vi "2_test_1.vi"() -> ()   [LabVIEW 2020]
uses:
  <vilib>/vision/driver/NI_Vision_Acquisition_Software.lvlib
panel:
  out "error out":errorcluster
  in  "停止":bool
  in  "error in":errorcluster
  in  "File Path":path
  in  "Session In":refnum<k21>
  out "Image":T1(plugin-control)
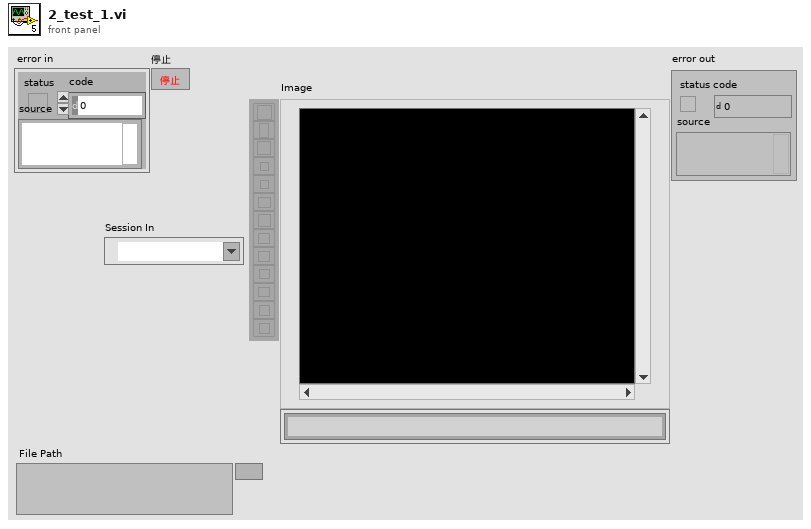
[diagram p1: front panel]
types:
  T1 = typedef "IMAQ Image.ctl" = refnum<image>
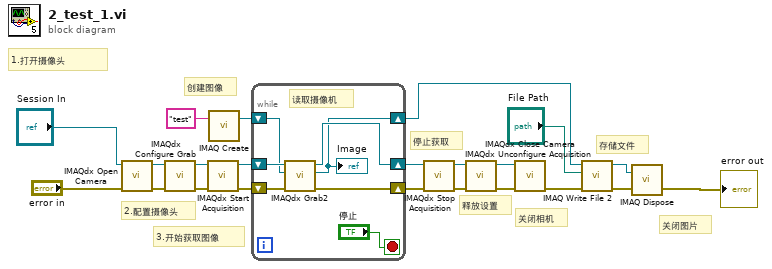
[diagram p0: block diagram]
diagram:
  # "关闭图片"
  # "存储文件"
  # "关闭相机"
  # "释放设置"
  # "停止获取"
  # "创建图像"
  # "3.开始获取图像"
  # "2.配置摄像头"
  # "1.打开摄像头"
  n1 = call <vilib>:"IMAQdx Open Camera.vi"("error in"="error in", "Session In"="Session In") -> ("error out"=w17:errorcluster, "Session Out"=w22:refnum<k21>)  [unwired: 8 in]
  n2 = call <vilib>:"IMAQdx Configure Grab.vi"("error in"=w17, "Session In"=w22) -> ("error out"=w18:errorcluster, "Session Out"=w20:refnum<k21>)  [unwired: 8 in]
  n3 = call <vilib>:"IMAQdx Start Acquisition.vi"("error in"=w18, "Session In"=w20) -> ("error out"=w19:errorcluster, "Session Out"=w21:refnum<k21>)  [unwired: 8 in]
  n4 = call "IMAQ Create"("Image Name"="test") -> ("New Image"=w10:T1)  [unwired: 4 in, 1 out]
  n5 = while {
    shift-right: [w27] -> w15
    shift-left: w21 -> [w29]
    shift-right: [w26] -> w16
    shift-left: w19 -> [w28]
    shift-right: [w23] -> w8
    shift-left: w10 -> [w25]
    stop <- "停止" stop-if-true
    # "读取摄像机"
    n6 = call <vilib>:"IMAQdx Grab2.vi"("error in"=w28, "Image In"=w25, "Session In"=w29) -> ("error out"=w26:errorcluster, "Image Out"=w23:T1, "Session Out"=w27:refnum<k21>)  [unwired: 5 in, 1 out]
    "Image" <- w23
  }
  n7 = call <vilib>:"IMAQdx Stop Acquisition.vi"("error in"=w16, "Session In"=w15) -> ("error out"=w5:errorcluster, "Session Out"=w7:refnum<k21>)  [unwired: 8 in]
  n8 = call <vilib>:"IMAQdx Unconfigure Acquisition.vi"("error in"=w5, "Session In"=w7) -> ("error out"=w4:errorcluster, "Session Out"=w6:refnum<k21>)  [unwired: 8 in]
  n9 = call <vilib>:"IMAQdx Close Camera.vi"("error in"=w4, "Session In"=w6) -> ("error out"=w14:errorcluster)  [unwired: 9 in]
  n10 = call-poly "IMAQ Write File 2"("error in (no error)"=w14, "File Path"="File Path", "Image"=w8) -> ("error out"=w2:errorcluster, "Image Out (duplicate)"=w3:T1)  [unwired: 7 in]
  n11 = call "IMAQ Dispose"("Image"=w3, "error in (no error)"=w2) -> ("error out"=→"error out":errorcluster)  [unwired: 4 in]
